vi "Patch_Multipart_Method.vi"(6 "Headers":cluster{"Name":string, "Value":string}[](array[cluster]), 8 "error in (no error)":errorcluster, 9 "Multpart/Form-Data":T1(array[cluster]), 10 "Endpoint URL":string, 11 "Request in":refnum<class "Request.lvclass">) -> (0 "error out":errorcluster, 2 "Response out":refnum<class "Response.lvclass">, 3 "Request out":refnum<class "Request.lvclass">)   [LabVIEW 2016]
uses:
  Request/Request.lvclass
  Response/Response.lvclass
  Request/PowerShell_Format/Request_Control.ctl
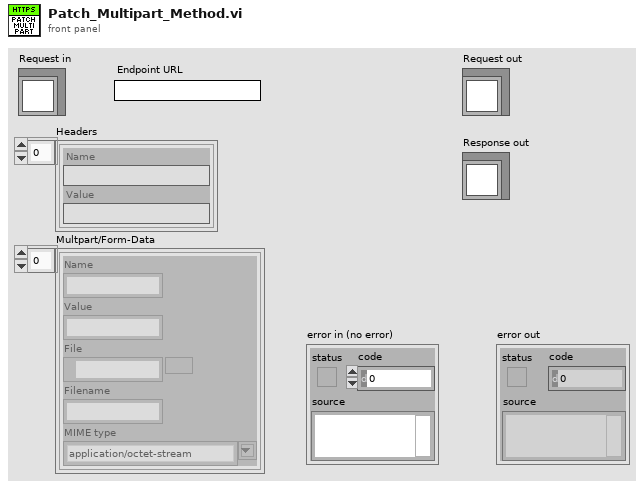
[diagram p1: front panel]
types:
  T1 = cluster{"Name":string, "Value":string, "File":path, "Filename":string, "MIME type":string}[]
  T2 = typedef "Request.lvclass/Request_Control.ctl" = enum16{"POST", "PATCH_MULTIPART", "POST_MULTIPART", "PATCH", "DELETE", "HEAD", "PUT", "GET"}
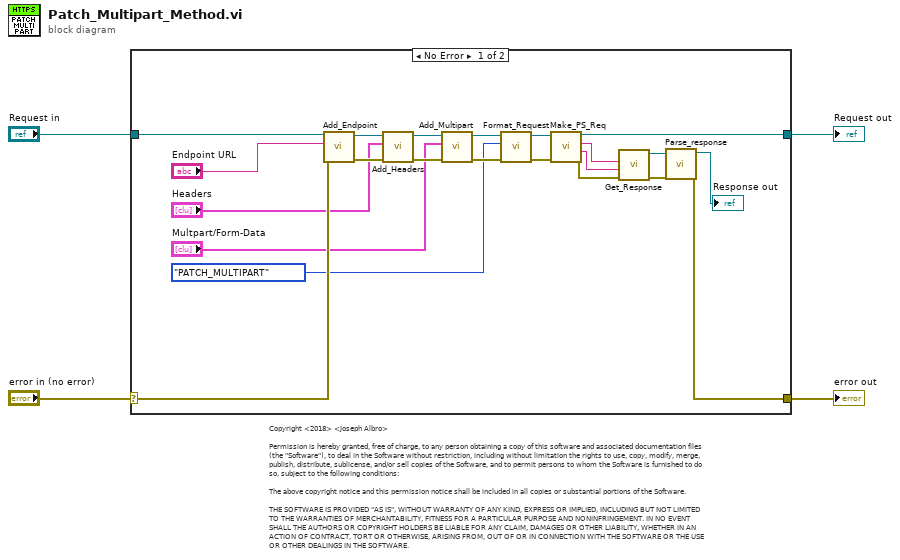
[diagram p0: block diagram]
diagram:
  # "Copyright <2018> <Joseph Albro>\n\nPermission is hereby granted, free of charge, to any person obtaining a copy of this software and associated documentation files (the \"Software\"), to deal in the Software without restriction, including without limitation the rights to use, copy, modify, merge, publish, distribute, sublicense, and/or sell copies of the Software, and to permit persons to whom the Software is furnished to do so, subject to the following conditions:\n\nThe above copyright notice and this permission notice shall be included in all copies or substantial portions of the Software.\n\nTHE SOFTWARE IS PROVIDED \"AS IS\", WITHOUT WARRANTY OF ANY KIND, EXPRESS OR IMPLIED, INCLUDING BUT NOT LIMITED TO THE WARRANTIES OF MERCHANTABILITY, FITNESS FOR A PARTICULAR PURPOSE AND NONINFRINGEMENT. IN NO EVENT SHALL THE AUTHORS OR COPYRIGHT HOLDERS BE LIABLE FOR ANY CLAIM, DAMAGES OR OTHER LIABILITY, WHETHER IN AN ACTION OF CONTRACT, TORT OR OTHERWISE, ARISING FROM, OUT OF OR IN CONNECTION WITH THE SOFTWARE OR THE USE OR OTHER DEALINGS IN THE SOFTWARE."
  n1 = case shown="No Error" "error in (no error)" {
    selector: "error in (no error)" -> [w10 w28]
    tunnel: [w9 w28] -> w3
    tunnel: [w20 w27] -> w1
    tunnel: "Request in" -> [w23 w27]
    frame No Error {
      n2 = call "Add_Endpoint.vi"("error in (no error)"=w10, "Endpoint URL"="Endpoint URL", "Request in"=w23) -> ("error out"=w11:errorcluster, "Request out"=w26:refnum<class "Request.lvclass">)  [unwired: 7 in]
      n3 = call "Add_Headers.vi"("error in (no error)"=w11, "Headers"="Headers", "Request in"=w26) -> ("error out"=w12:errorcluster, "Request out"=w25:refnum<class "Request.lvclass">)  [unwired: 7 in]
      n4 = call "Add_Multipart.vi"("error in (no error)"=w12, "Multpart/Form-Data"="Multpart/Form-Data", "Request in"=w25) -> ("error out"=w13:errorcluster, "Request out"=w24:refnum<class "Request.lvclass">)  [unwired: 7 in]
      n5 = call "Format_Request.vi"("error in (no error)"=w13, "Request"=Request_Control."PATCH_MULTIPART", "Request in"=w24) -> ("error out"=w14:errorcluster, "Request out"=w21:refnum<class "Request.lvclass">)  [unwired: 7 in]
      n6 = call "Make_PS_Req.vi"("error in (no error)"=w14, "Request in"=w21) -> ("error out"=w15:errorcluster, "standard error"=w18:string, "standard output"=w19:string, "Request out"=w20:refnum<class "Request.lvclass">)  [unwired: 6 in]
      n7 = call "Get_Response.vi"("error in (no error)"=w15, "PS Error"=w18, "PS Response"=w19) -> ("error out"=w16:errorcluster, "Response out"=w17:refnum<class "Response.lvclass">)  [unwired: 7 in]
      n8 = call "Parse_response.vi"("error in (no error)"=w16, "Response in"=w17) -> ("error out"=w9:errorcluster, "Response out"=→"Response out":refnum<class "Response.lvclass">)  [unwired: 8 in]
    }
    frame Error {
    }
  }
  "error out" <- w3
  "Request out" <- w1
